vi "GetRingRef.vi"(11 "Array Reference":refnum<vi>) -> (0 "error out":errorcluster, 3 "Ring Reference":refnum<vi>)   [LabVIEW 2016]
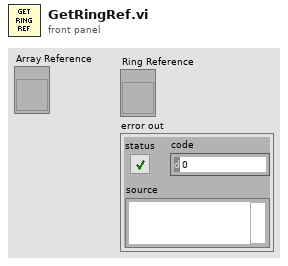
[diagram p1: front panel]
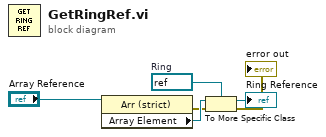
[diagram p0: block diagram]
diagram:
  w5 = refnum<vi> refnum  # Ring
  n1 = property class="Arr (strict)"(reference="Array Reference") -> (error out=w4:errorcluster, "Array Element"=w6:refnum<vi>)  [unwired: 1 in, 1 out]
  n2 = To More Specific Class(target class=w5, reference=w6, error in=w4) -> (specific class reference=→"Ring Reference":refnum<vi>, error out=→"error out":errorcluster)
